vi "writeITC503control_channel.vi"(3 "Control Channel":i16, 5 "ITC IO Info 2":T1={"Com Port"=1, "ISOBUS Address"=1, "GPIB Address"=1, "Communication"=enum."ISOBUS"}) -> (2 "ITC IO Info":T1={"Com Port"=1, "ISOBUS Address"=1, "GPIB Address"=1, "Communication"=enum."ISOBUS"})   [LabVIEW 2019]
uses:
  Equipment/Oxford Software/Oxsoft/ITCSUBS.LLB/ITCIO.ctl
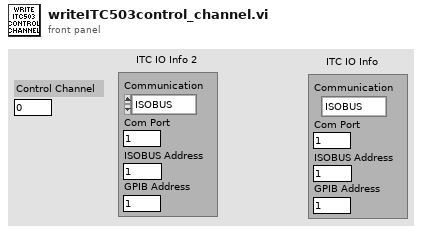
[diagram p1: front panel]
types:
  T1 = typedef "ITCIO.ctl" = cluster{"Com Port":i32, "ISOBUS Address":i32, "GPIB Address":i16, "Communication":enum16{"RS232", "ISOBUS", "GPIB", "Gateway"}}
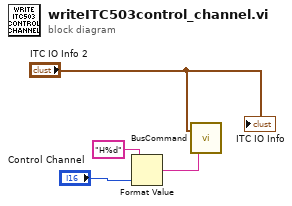
[diagram p0: block diagram]
diagram:
  n1 = Format Value(format string="H%d", value (0)="Control Channel") -> (output string=w4:string)  [unwired: 1 in]
  n2 = call "BusCommand.vi"("Command"=w4, "Instrument address (in)"="ITC IO Info 2") -> ()  [unwired: 2 out]
  "ITC IO Info" <- "ITC IO Info 2"
